vi "Load Firebase Info.vi"(8 "error in":errorcluster, 9 "Firebase URL":string="https://samdemo-e0b7e-default-rtdb.firebaseio.com/", 10 "API_KEY":string="AIzaSyCG-sCHoMequsURAUDnZonTKWK1rmJvs14", 11 "firebase in":refnum<class "firebase.lvclass">) -> (0 "error out":errorcluster, 3 "firebase out":refnum<class "firebase.lvclass">)   [LabVIEW 2019, in "firebase.lvclass"]
uses:
  firebase.lvclass
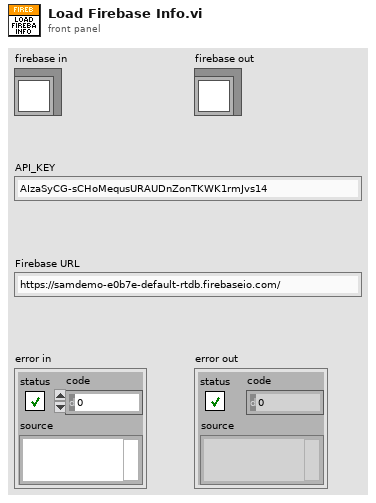
[diagram p1: front panel]
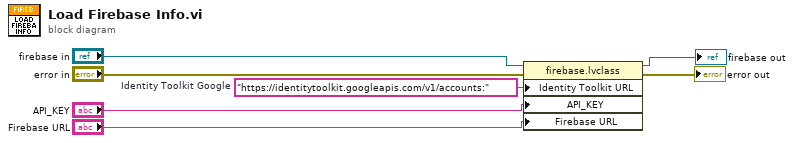
[diagram p0: block diagram]
diagram:
  w3 = "https://identitytoolkit.googleapis.com/v1/accounts:"  # Identity Toolkit Google
  n1 = property class="firebase.lvclass"(reference="firebase in", error in="error in", "Identity Toolkit URL"=w3, "API_KEY"="API_KEY", "Firebase URL"="Firebase URL") -> (reference out=→"firebase out":refnum<class "firebase.lvclass">, error out=→"error out":errorcluster)
